vi "build.vi"(8 "error in (no error)":errorcluster, 10 "Package?":bool=TRUE, 11 "Build?":bool=TRUE) -> (0 "error out":errorcluster)   [LabVIEW 2017]
uses:
  <vilib>/Utility/config.llb/Read Key (String).vi
  <vilib>/Utility/config.llb/NI_LVConfig.lvlib
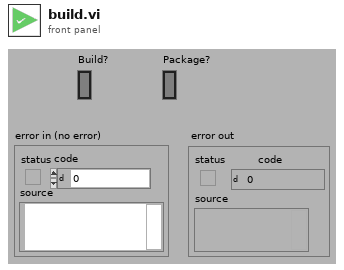
[diagram p1: front panel]
types:
  T1 = typedef "NI_LVConfig.lvlib/Config Data RefNum.ctl" = refnum<k1>
  T2 = typedef "OGPM Package Spec__ogpb_api.ctl" = cluster{"Package Name":T3, "Platform":T4, "File Groups":T6[], "Description":T7, "Files":T8, "Script VIs":T9, "Dependencies":T10}
  T3 = typedef "OGPM Spec - Package Name - Cluster__ogpb_api.ctl" = cluster{"Name":string, "Version":string, "Release":string}
  T4 = typedef "OGPM Package Spec Platform__ogpb_api.ctl" = cluster{"Exclusive_LabVIEW_Version":cluster{"Comparison":enum16{">=", "<=", ">", "<", "="}, "Version":u8[]}[], "Exclusive_LabVIEW_System":string[], "Exclusive_OS":T5[], "Exclude_LabVIEW_Version":cluster{"Comparison":enum16{">=", "<=", ">", "<", "="}, "Version":u8[]}[], "Exclude_OS":T5[], "Exclude_LabVIEW_System":string[]}
  T5 = typedef "OGPM OS Dependency Cluster__ogpb_api.ctl" = cluster{"OS Name":string, "Comparison":enum16{">=", "<=", ">", "<", "="}, "Version":u8[]}
  T6 = typedef "OGPM Package - File Group - Cluster__ogpb_api.ctl" = cluster{"Source Dir":path, "Target Dir":path, "Replace Mode":enum16{"Never", "Always", "If Newer"}, "Num Files":u32, "Files":path[], "Exclusive_LabVIEW_Version":cluster{"Comparison":enum16{">=", "<=", ">", "<", "="}, "Version":u8[]}[], "Exclusive_OS":T5[], "Exclusive_LabVIEW_System":string[], "Exclude_LabVIEW_Version":cluster{"Comparison":enum16{">=", "<=", ">", "<", "="}, "Version":u8[]}[], "Exclude_OS":T5[], "Exclude_LabVIEW_System":string[]}
  T7 = typedef "OGPM Spec - Description - Cluster__ogpb_api.ctl" = cluster{"Description":string, "Summary":string, "License":string, "Copyright":string, "Distribution":string, "Icon":path, "Vendor":string, "URL":string, "Packager":string}
  T8 = typedef "OGPM Package - Files - Cluster__ogpb_api.ctl" = cluster{"Source Dir":path, "Target Dir":path, "Num File Groups":u32, "Documentation":string, "Doc Groups":u32[]}
  T9 = typedef "OGPM Package Spec Script VIs__ogpb_api.ctl" = cluster{"Source Dir":path, "PreInstall":string, "PostInstall":string, "PreUninstall":string, "PostUninstall":string, "Verify":string, "PreBuild":string, "PostBuild":string}
  T10 = typedef "OGPM Package Spec Dependencies__ogpb_api.ctl" = cluster{"Depends":T11[], "Conflicts":T11[], "AutoReqProv":bool}
  T11 = typedef "OGPM Package Dependency Cluster__ogpb_api.ctl" = cluster{"Pkg Name":string, "Comparison":enum16{">=", "<=", ">", "<", "="}, "Version":u8[]}
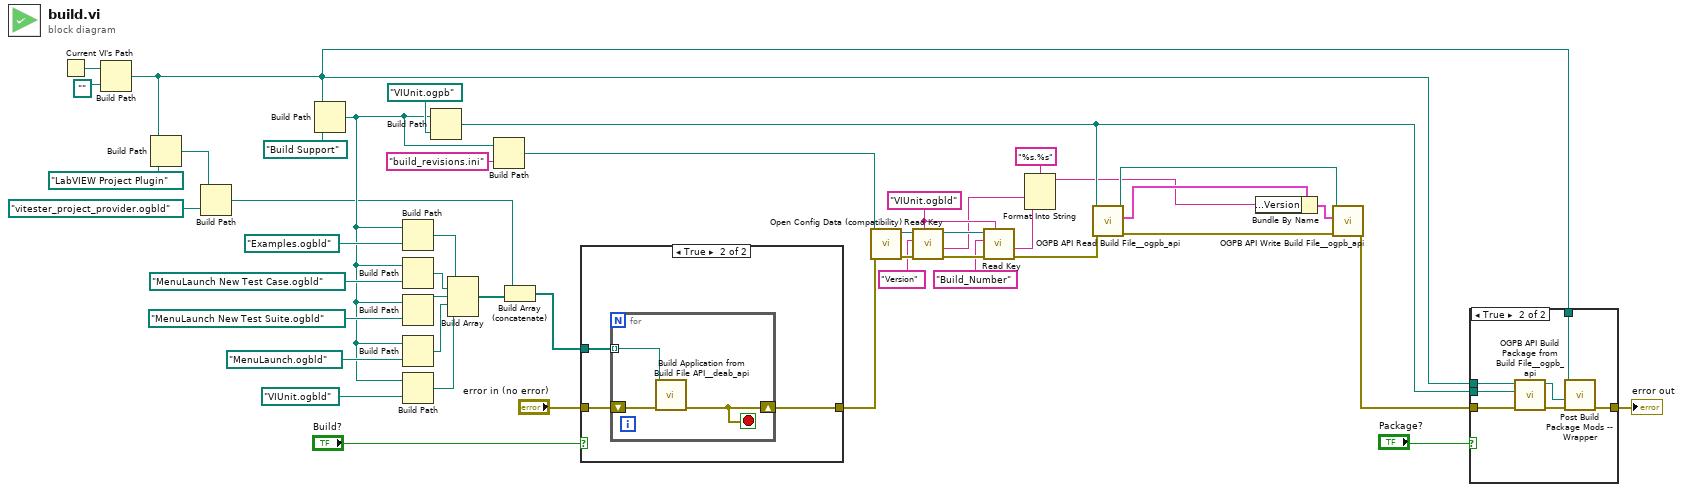
[diagram p0: block diagram]
diagram:
  w26 = "VIUnit.ogbld" ("section")
  n1 = Current VI's Path() -> (path=w47:path)
  n2 = Build Path(base path=w47, name or relative path=path ".." ("base path")) -> (appended path=w7:path)
  n3 = Build Path(base path=w7, name or relative path=path "LabVIEW Project Plugin" ("base path")) -> (appended path=w4:path)
  n4 = Build Path(base path=w4, name or relative path=path "vitester_project_provider.ogbld") -> (appended path=w1:path)
  n5 = Build Path(base path=w7, name or relative path=path "Build Support" ("base path")) -> (appended path=w8:path)
  n6 = Build Path(base path=w8, name or relative path=path "Examples.ogbld" ("base path")) -> (appended path=w33:path)
  n7 = Build Path(base path=w8, name or relative path=path "MenuLaunch New Test Case.ogbld" ("base path")) -> (appended path=w35:path)
  n8 = Build Path(base path=w8, name or relative path=path "MenuLaunch New Test Suite.ogbld" ("base path")) -> (appended path=w9:path)
  n9 = Build Path(base path=w8, name or relative path=path "MenuLaunch.ogbld" ("base path")) -> (appended path=w36:path)
  n10 = Build Path(base path=w8, name or relative path=path "VIUnit.ogbld" ("base path")) -> (appended path=w37:path)
  n11 = Build Path(base path=w8, name or relative path=path "VIUnit.ogpb" ("base path")) -> (appended path=w20:path)
  n12 = Build Array(w33, w35, w9, w36, w37) -> (w3:path[])
  n13 = Build Path(base path=w8, name or relative path="build_revisions.ini") -> (appended path=w24:path)
  n14 = Build Array (concatenate)(w1, w3) -> (w2:path[])
  n15 = case shown="True" "Build?" {
    tunnel: [_ w49] -> w23
    tunnel: w2 -> [_ w50]
    tunnel: "error in (no error)" -> [_ w48]
    frame False {
    }
    frame True {
      n16 = for {
        tunnel: w50 -> [w52] mode=indexing
        shift-right: [w51] -> w49
        shift-left: w48 -> [w53]
        stop <- w51 stop-if-true
        n17 = call <userlib>:"Build Application from Build File API__deab_api.vi"("error in (no error)"=w53, "Build file path"=w52) -> ("error out"=w51:errorcluster)  [unwired: 8 in, 1 out]
      }
    }
  }
  n18 = call <vilib>:"Open Config Data (compatibility).vi"("error in (no error)"=w23, "configuration file path"=w24) -> ("error out"=w30:errorcluster, "refnum"=w29:T1)  [unwired: 7 in, 1 out]
  n19 = call-poly <vilib>:"Read Key.vi"("section"=w26, "error in (no error)"=w30, "key"="Version", "refnum"=w29) -> ("error out"=w27:errorcluster, "value"=w17:string, "refnum out"=w28:T1)  [unwired: 4 in, 1 out]
  n20 = call-poly <vilib>:"Read Key.vi"("section"=w26, "error in (no error)"=w27, "key"="Build_Number", "refnum"=w28) -> ("error out"=w13:errorcluster, "value"=w16:string)  [unwired: 4 in, 2 out]
  n21 = Format Into String(format string="%s.%s", w17, w16) -> (resulting string=w14:string)  [unwired: 2 in, 1 out]
  n22 = call <userlib>:"OGPB API Read Build File__ogpb_api.vi"("error in (no error)"=w13, "Build File path"=w20) -> ("error out"=w18:errorcluster, "Spec out"=w22:T2, "dup Build File path"=w19:path)  [unwired: 7 in]
  n23 = Bundle By Name(cluster=w22, "Package Name.Version"=w14) -> (w21:T2)
  n24 = call <userlib>:"OGPB API Write Build File__ogpb_api.vi"("error in (no error)"=w18, "Spec in"=w21, "Build File path"=w19) -> ("error out"=w12:errorcluster)  [unwired: 7 in, 1 out]
  n25 = case shown="True" "Package?" {
    tunnel: w12 -> [w54 w55]
    tunnel: w7 -> [_ w61]
    tunnel: [w54 w59] -> w40
    tunnel: w20 -> [_ w56]
    tunnel: w7 -> [_ w57]
    frame False {
    }
    frame True {
      n26 = call <userlib>:"OGPB API Build Package from Build File__ogpb_api.vi"("error in (no error)"=w55, "Build File path"=w56, "Package Dest Dir"=w61) -> ("error out"=w60:errorcluster, "Built package path"=w58:path)  [unwired: 7 in]
      n27 = call "Post Build Package Mods -- Wrapper.vi"("error in (no error)"=w60, "Built package path"=w58, "Project Root"=w57) -> ("error out"=w59:errorcluster)  [unwired: 8 in]
    }
  }
  "error out" <- w40
